vi "Operational Force Test DAA.vi"(8 "error in (no error)":errorcluster, 10 "Model in":refnum<class "Model.lvclass">, 11 "Test Actuator State in":refnum<class "Test Actuator State.lvclass">) -> (0 "error out":errorcluster, 1 "Pass":bool, 2 "Model out":refnum<class "Model.lvclass">, 3 "Test Actuator State out":refnum<class "Test Actuator State.lvclass">)   [LabVIEW 2016]
uses:
  Model/Model/Model.lvclass
  Typedefs/ActuatorSetPoints.ctl
  <vilib>/platform/TimedLoop/XDataNode/XDataNode.xnode
  <vilib>/Platform/TimedLoop/XDataNode/nitl_modes.ctl
  <vilib>/Platform/TimedLoop/XDataNode/XDNodeRunTimeDep.lvlib
  <vilib>/Platform/TimedLoop/XDataNode/wakeup.ctl
  <vilib>/Platform/TimedLoop/XDataNode/timing_clust.ctl
  Test Actuator State.lvclass
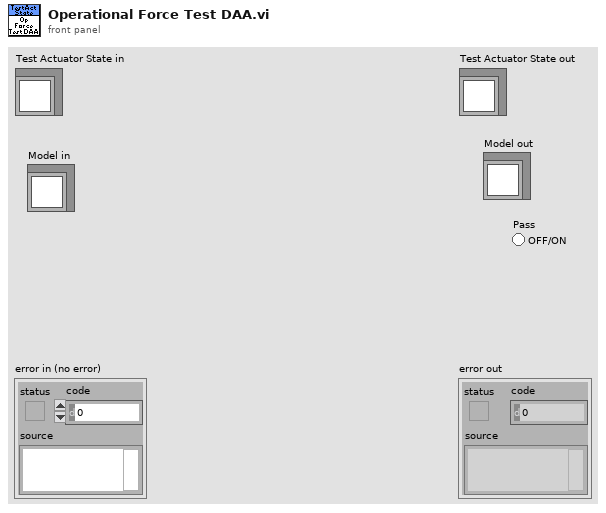
[diagram p1: front panel]
types:
  T1 = typedef "ForcePair.ctl" = cluster{"Axial Force":dbl, "Lateral Force":dbl}
  T2 = typedef "OperationalForceTestSettings.ctl" = cluster{"Max Force Error (N)":dbl, "Max Moment (NM)":dbl, "Process Time (s)":dbl, "Sample Time (s)":dbl}
  T3 = typedef "ActuatorSetPoints.ctl" = cluster{"Axial Force":dbl, "Lateral Force":dbl, "FC1 Force":dbl, "FC2 Force":dbl}
  T4 = typedef "XDNodeRunTimeDep.lvlib/timing_clust.ctl" = cluster{"Expected End [f-1]":u64, "Actual End [f-1]":u64, "Finished Late? [f-1]":bool, "Expected End [i-1]":u64, "Actual End [i-1]":u64, "Finished Late? [i-1]":bool, "Expected Start [i]":u64, "Actual Start [i]":u64, "Expected Start [f]":u64, "Actual Start [f]":u64, "Source Name":string, "Structure Name":string, "Period":i64, "Deadline":i64, "Offset":i64, "Start":i64, "Priority":i32, "Timeout":i32, "Mode":T5, "Wakeup Reason":T6, "Error":errorcluster, "Source Type":string, "Secondary Source Type":string, "Global End Time":u64, "Global Start Time":u64, "Frame Duration":u64, "Iteration Duration":u64, "Assigned CPU":i32, "I/O Scan Engine Mode":u32}
  T5 = typedef "XDNodeRunTimeDep.lvlib/nitl_modes.ctl" = enum32{"No Change", "Process missed periods, maintain original phase", "Discard missed periods, maintain original phase", "Process missed periods, ignore original phase", "Discard missed periods, ignore original phase"}
  T6 = typedef "XDNodeRunTimeDep.lvlib/wakeup.ctl" = enum32{"Normal", "Aborted", "Asynchronous wakeup", "Timing source error", "Timed loop error", "Timeout"}
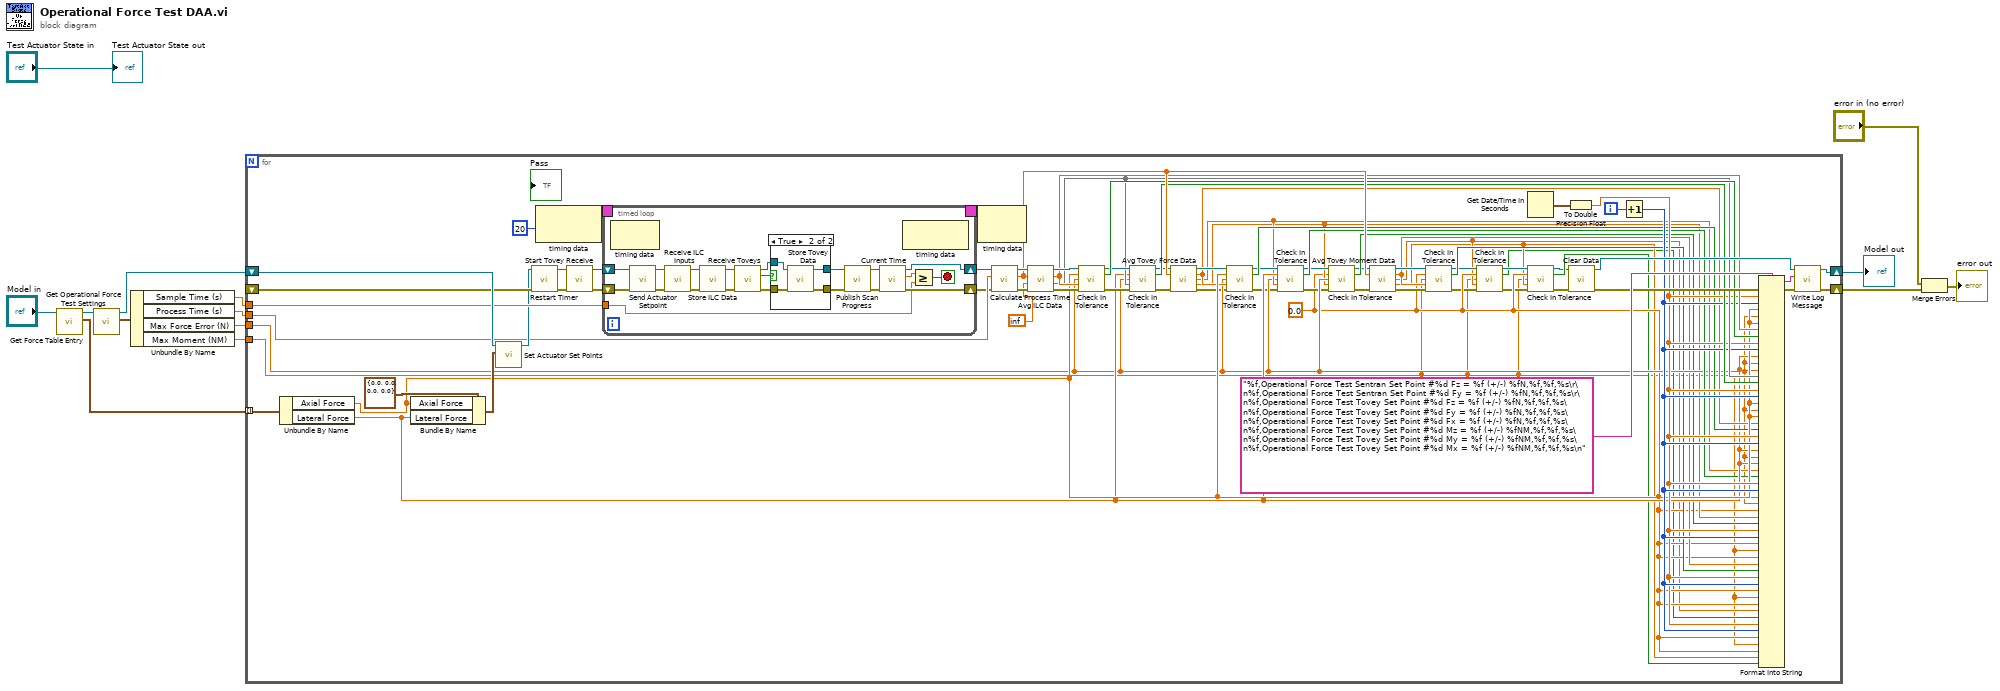
[diagram p0: block diagram]
diagram:
  n1 = call "Get Force Table Entry.vi"("Model in"="Model in") -> ("Entry"=w1:T1[], "Model out"=w4:refnum<class "Model.lvclass">)  [unwired: 8 in, 1 out]
  n2 = call-dynamic "Get Operational Force Test Settings.vi"("Model in"=w4) -> ("Operational Force Test Settings"=w2:T2, "Model out"=w3:refnum<class "Model.lvclass">)  [unwired: 9 in]
  n3 = Unbundle By Name(w2) -> ("Sample Time (s)"=w13:dbl, "Process Time (s)"=w12:dbl, "Max Force Error (N)"=w11:dbl, "Max Moment (NM)"=w6:dbl)
  n4 = for {
    tunnel: w1 -> [w74] mode=indexing
    shift-right: [w84] -> w8
    shift-left: w3 -> [w88]
    tunnel: w13 -> [w87]
    tunnel: w12 -> [w69]
    tunnel: w11 -> [w42]
    shift-right: [w70] -> w7
    shift-left: _ -> [w86]
    tunnel: w6 -> [w19]
    i -> [w81]
    w28 = 0.0
    n5 = Unbundle By Name(w74) -> ("Axial Force"=w50:dbl, "Lateral Force"=w46:dbl)
    n6 = Bundle By Name(cluster=T3 {"Axial Force"=0.0, "Lateral Force"=0.0, "FC1 Force"=0.0, "FC2 Force"=0.0} ("Actuator Set Points"), "Axial Force"=w50, "Lateral Force"=w46) -> (w75:T3)
    n7 = call "Set Actuator Set Points.vi"("Actuator Set Points"=w75, "Model in"=w88) -> ("Model out"=w76:refnum<class "Model.lvclass">)  [unwired: 9 in]
    n8 = call "Restart Timer.vi"("error in (no error)"=w86, "Model in"=w76) -> ("error out"=w79:errorcluster, "Model out"=w80:refnum<class "Model.lvclass">)  [unwired: 8 in]
    n9 = node-c288(i64 20 ("Period")) -> (w17:T4)
    n10 = call "Start Tovey Receive.vi"("error in (no error)"=w79, "Model in"=w80) -> ("error out"=w77:errorcluster, "Model out"=w78:refnum<class "Model.lvclass">)  [unwired: 8 in]
    n11 = timed-loop {
      shift-right: [w103] -> w68
      shift-left: w78 -> [w109]
      shift-right: [w102] -> w66
      shift-left: w77 -> [w106]
      tunnel: w87 -> [w100]
      timing: w17 -> [_]
      timing-out: [_] -> w16
      stop <- w99 stop-if-true
      n12 = node-c288() -> ()  [unwired: 1 in, 1 out]
      n13 = call "Send Actuator Setpoint.vi"("error in (no error)"=w106, "Model in"=w109) -> ("error out"=w105:errorcluster, "Model out"=w108:refnum<class "Model.lvclass">)  [unwired: 8 in]
      n14 = call "Receive ILC Inputs.vi"("error in (no error)"=w105, "Model in"=w108) -> ("error out"=w104:errorcluster, "Model out"=w107:refnum<class "Model.lvclass">)  [unwired: 8 in]
      n15 = call "Store ILC Data.vi"("error in (no error)"=w104, "Model in"=w107) -> ("error out"=w97:errorcluster, "Model out"=w98:refnum<class "Model.lvclass">)  [unwired: 8 in]
      n16 = call "Receive Toveys.vi"("error in (no error)"=w97, "Model in"=w98) -> ("error out"=w95:errorcluster, "Data Received"=w94:bool, "Model out"=w96:refnum<class "Model.lvclass">)  [unwired: 7 in]
      n17 = case shown="True" w94 {
        tunnel: w96 -> [w113 w117]
        tunnel: w95 -> [w112 w116]
        tunnel: [w112 w115] -> w90
        tunnel: [w113 w114] -> w93
        frame False {
        }
        frame True {
          n18 = call "Store Tovey Data.vi"("error in (no error)"=w116, "Model in"=w117) -> ("error out"=w115:errorcluster, "Model out"=w114:refnum<class "Model.lvclass">)  [unwired: 8 in]
        }
      }
      n19 = call "Publish Scan Progress.vi"("error in (no error)"=w90, "Model in"=w93) -> ("error out"=w91:errorcluster, "Model out"=w92:refnum<class "Model.lvclass">)  [unwired: 8 in]
      n20 = call "Current Time.vi"("error in (no error)"=w91, "Model in"=w92) -> ("error out"=w102:errorcluster, "Time"=w101:dbl, "Model out"=w103:refnum<class "Model.lvclass">)  [unwired: 7 in]
      n21 = node-c288() -> ()  [unwired: 1 in, 1 out]
      n22 = Greater Or Equal?(x=w101, y=w100) -> (x >= y?=w99:bool)
    }
    n23 = node-c288(w16) -> ()  [unwired: 1 out]
    n24 = call "Calculate Process Time.vi"("error in (no error)"=w66, "Seconds"=w69, "Model in"=w68) -> ("error out"=w65:errorcluster, "Time"=w64:dbl, "Model out"=w67:refnum<class "Model.lvclass">)  [unwired: 6 in]
    n25 = call "Avg ILC Data.vi"("error in (no error)"=w65, "Before This Time"=inf, "After This Time"=w64, "Model in"=w67) -> ("error out"=w57:errorcluster, 1:w59, "Force"=w62:dbl, "Model out"=w63:refnum<class "Model.lvclass">)  [unwired: 4 in]
    n26 = call "Check In Tolerance.vi"("Model in"=w63, "Expected"=w50, "Tolerance"=w42, "Actual"=w62, "error in (no error)"=w57) -> ("Model out"=w60:refnum<class "Model.lvclass">, "Pass"=w61:bool, "error out"=w56:errorcluster)  [unwired: 8 in]
    n27 = call "Check In Tolerance.vi"("Model in"=w60, "Expected"=w46, "Tolerance"=w42, "Actual"=w59, "error in (no error)"=w56) -> ("Model out"=w54:refnum<class "Model.lvclass">, "Pass"=w58:bool, "error out"=w55:errorcluster)  [unwired: 8 in]
    n28 = call "Avg Tovey Force Data.vi"("Model in"=w54, "After This Time"=w64, "error in (no error)"=w55) -> ("Model out"=w51:refnum<class "Model.lvclass">, "Fz"=w48:dbl, "Fy"=w44:dbl, "Fx"=w32:dbl, "error out"=w39:errorcluster)  [unwired: 8 in]
    n29 = call "Check In Tolerance.vi"("Model in"=w51, "Expected"=w50, "Tolerance"=w42, "Actual"=w48, "error in (no error)"=w39) -> ("Model out"=w47:refnum<class "Model.lvclass">, "Pass"=w49:bool, "error out"=w38:errorcluster)  [unwired: 8 in]
    n30 = call "Check In Tolerance.vi"("Model in"=w47, "Expected"=w46, "Tolerance"=w42, "Actual"=w44, "error in (no error)"=w38) -> ("Model out"=w43:refnum<class "Model.lvclass">, "Pass"=w45:bool, "error out"=w37:errorcluster)  [unwired: 8 in]
    n31 = call "Check In Tolerance.vi"("Model in"=w43, "Expected"=w28, "Tolerance"=w42, "Actual"=w32, "error in (no error)"=w37) -> ("Model out"=w35:refnum<class "Model.lvclass">, "Pass"=w41:bool, "error out"=w36:errorcluster)  [unwired: 8 in]
    n32 = call "Avg Tovey Moment Data.vi"("Model in"=w35, "After This Time"=w64, "error in (no error)"=w36) -> ("Model out"=w34:refnum<class "Model.lvclass">, "Mz"=w31:dbl, "My"=w27:dbl, "Mx"=w26:dbl, "error out"=w33:errorcluster)  [unwired: 8 in]
    n33 = call "Check In Tolerance.vi"("Model in"=w34, "Expected"=w28, "Tolerance"=w19, "Actual"=w31, "error in (no error)"=w33) -> ("Model out"=w30:refnum<class "Model.lvclass">, "Pass"=w40:bool, "error out"=w22:errorcluster)  [unwired: 8 in]
    n34 = call "Check In Tolerance.vi"("Model in"=w30, "Expected"=w28, "Tolerance"=w19, "Actual"=w27, "error in (no error)"=w22) -> ("Model out"=w29:refnum<class "Model.lvclass">, "Pass"=w25:bool, "error out"=w21:errorcluster)  [unwired: 8 in]
    n35 = Get Date/Time In Seconds() -> (seconds since 1Jan1904=w82:timestamp)
    n36 = call "Check In Tolerance.vi"("Model in"=w29, "Expected"=w28, "Tolerance"=w19, "Actual"=w26, "error in (no error)"=w21) -> ("Model out"=w23:refnum<class "Model.lvclass">, "Pass"=w24:bool, "error out"=w20:errorcluster)  [unwired: 8 in]
    n37 = To Double Precision Float(number=w82) -> (double precision float=w52:dbl)
    n38 = call "Clear Data.vi"("error in (no error)"=w20, "Model in"=w23) -> ("error out"=w72:errorcluster, "Model out"=w85:refnum<class "Model.lvclass">)  [unwired: 8 in]
    n39 = Increment(x=w81) -> (x+1=w53:i32)
    n40 = Format Into String(format string="%f,Operational Force Test Sentran Set Point #%d Fz = %f (+/-) %fN,%f,%f,%s\r\n%f,Operational Force Test Sentran Set Point #%d Fy = %f (+/-) %fN,%f,%f,%s\r\n%f,Operational Force Test Tovey Set Point #%d Fz = %f (+/-) %fN,%f,%f,%s\n%f,Operational Force Test Tovey Set Point #%d Fy = %f (+/-) %fN,%f,%f,%s\n%f,Operational Force Test Tovey Set Point #%d Fx = %f (+/-) %fN,%f,%f,%s\n%f,Operational Force Test Tovey Set Point #%d Mz = %f (+/-) %fNM,%f,%f,%s\n%f,Operational Force Test Tovey Set Point #%d My = %f (+/-) %fNM,%f,%f,%s\n%f,Operational Force Test Tovey Set Point #%d Mx = %f (+/-) %fNM,%f,%f,%s\n", error in=w72, w52, w53, w50, w42, w50, w62, w61, w52, w53, w46, w42, w46, w59, w58, w52, w53, w50, w42, w50, w48, w49, w52, w53, w46, w42, w46, w44, w45, w52, w53, w28, w42, w28, w32, w41, w52, w53, w28, w19, w28, w31, w40, w52, w53, w28, w19, w28, w27, w25, w52, w53, w28, w19, w28, w26, w24) -> (resulting string=w73:string, error out=w71:errorcluster)  [unwired: 1 in]
    n41 = call "Write Log Message.vi"("error in (no error)"=w71, "Message"=w73, "Model in"=w85) -> ("error out"=w70:errorcluster, "Model out"=w84:refnum<class "Model.lvclass">)  [unwired: 7 in]
  }
  "Model out" <- w8
  n42 = Merge Errors("error in (no error)", w7) -> (→"error out":errorcluster)
  "Test Actuator State out" <- "Test Actuator State in"
